vi "Set Controls(Axis).vi"(2 "Axis Actions Secondary":T1(ring), 3 "Axis Actions Primary":T2) -> (0 "Axis Secondary":dbl, 1 "Axis Primary":dbl)   [LabVIEW 2014]
uses:
  Axis Actions.ctl
  SRE Enum.ctl
  Support Code/Robot Global Data.vi
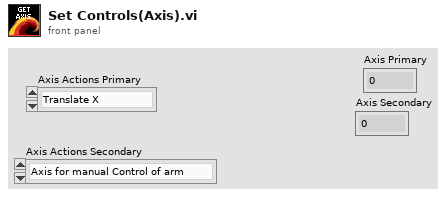
[diagram p1: front panel]
types:
  T1 = enum16{"Axis for manual Control of arm", "Axis for manual Control of Claw", "Rotate Claw"}
  T2 = typedef "Axis Actions.ctl" = enum16{"Translate X", "Translate Y", "Rotate"}
  T3 = typedef "SRE Enum.ctl" = enum16{"Start", "Run", "End"}
  T4 = enum16{"Left X", "Left Y", "Left trigger", "R trigger", "R X", "R Y"}[]
  T5 = enum16{"X left ", "Y left", "Z left", "X right", "Y right", "Z right"}[]
  T6 = enum16{"Left X", "Left Y", "Left trigger", "R trigger", "R X", "R Y"}
  T7 = enum16{"X left ", "Y left", "Z left", "X right", "Y right", "Z right"}
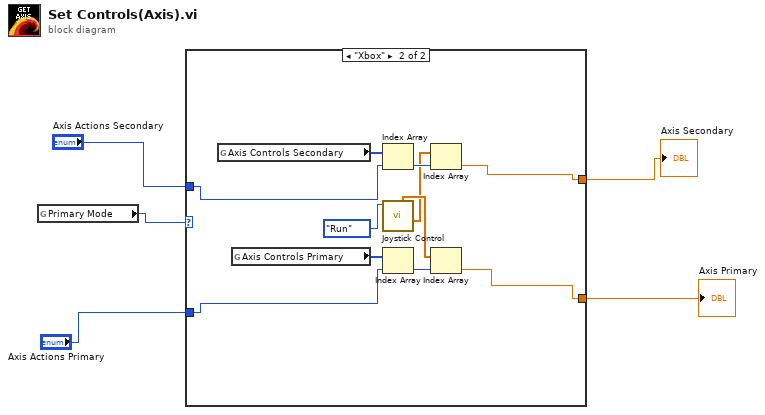
[diagram p0: block diagram]
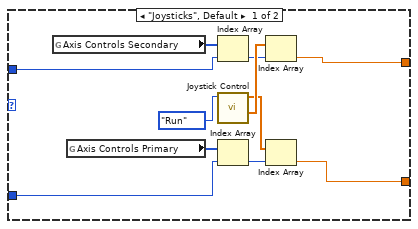
[diagram p2: hidden frame]
diagram:
  n1 = global read "Robot Global Data.vi" "Primary Mode"() -> (w5:enum16{"Joysticks", "Xbox"})
  n2 = case shown="\"Xbox\"" w5 {
    tunnel: [w9 w19] -> w4
    tunnel: [w8 w22] -> w3
    tunnel: "Axis Actions Primary" -> [w7 w20]
    tunnel: "Axis Actions Secondary" -> [w6 w21]
    frame "Joysticks", Default {
      n3 = global read "Robot Global Data.vi" "Axis Controls Secondary"() -> (w15:T4)
      n4 = global read "Robot Global Data.vi" "Axis Controls Primary"() -> (w11:T5)
      n5 = Index Array(array=w15, index=w6) -> (element=w13:T6)
      n6 = call "Joystick Control.vi"("Enum"=SRE_Enum."Run") -> ("Axis Output secondary"=w16:dbl[], "Axis Output PJ"=w10:dbl[])  [unwired: 3 in, 4 out]
      n7 = Index Array(array=w11, index=w7) -> (element=w12:T7)
      n8 = Index Array(array=w16, index=w13) -> (element=w8:dbl)
      n9 = Index Array(array=w10, index=w12) -> (element=w9:dbl)
    }
    frame "Xbox" {
      n10 = global read "Robot Global Data.vi" "Axis Controls Secondary"() -> (w23:T4)
      n11 = global read "Robot Global Data.vi" "Axis Controls Primary"() -> (w27:T5)
      n12 = Index Array(array=w23, index=w21) -> (element=w25:T6)
      n13 = call "Joystick Control.vi"("Enum"=SRE_Enum."Run") -> ("Axis Output secondary"=w17:dbl[], "Axis Output PX"=w18:dbl[])  [unwired: 3 in, 4 out]
      n14 = Index Array(array=w27, index=w20) -> (element=w26:T7)
      n15 = Index Array(array=w17, index=w25) -> (element=w22:dbl)
      n16 = Index Array(array=w18, index=w26) -> (element=w19:dbl)
    }
  }
  "Axis Secondary" <- w3
  "Axis Primary" <- w4
